vi "以太网测试界面.vi"() -> ()   [LabVIEW 2010]
panel:
  out "结果":bool
  out "接收数据":u32
  in  "发送数据":u32
  in  "btn_关闭":bool
  in  "btn_开始测试":bool
  # "以太网测试"
  # "输入数据："
  # "反馈数据："
  # "测试结果："
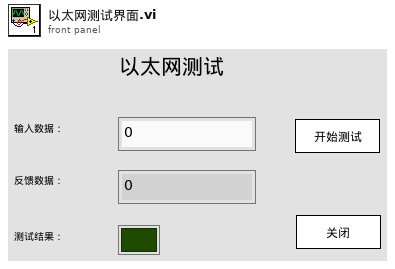
[diagram p1: front panel]
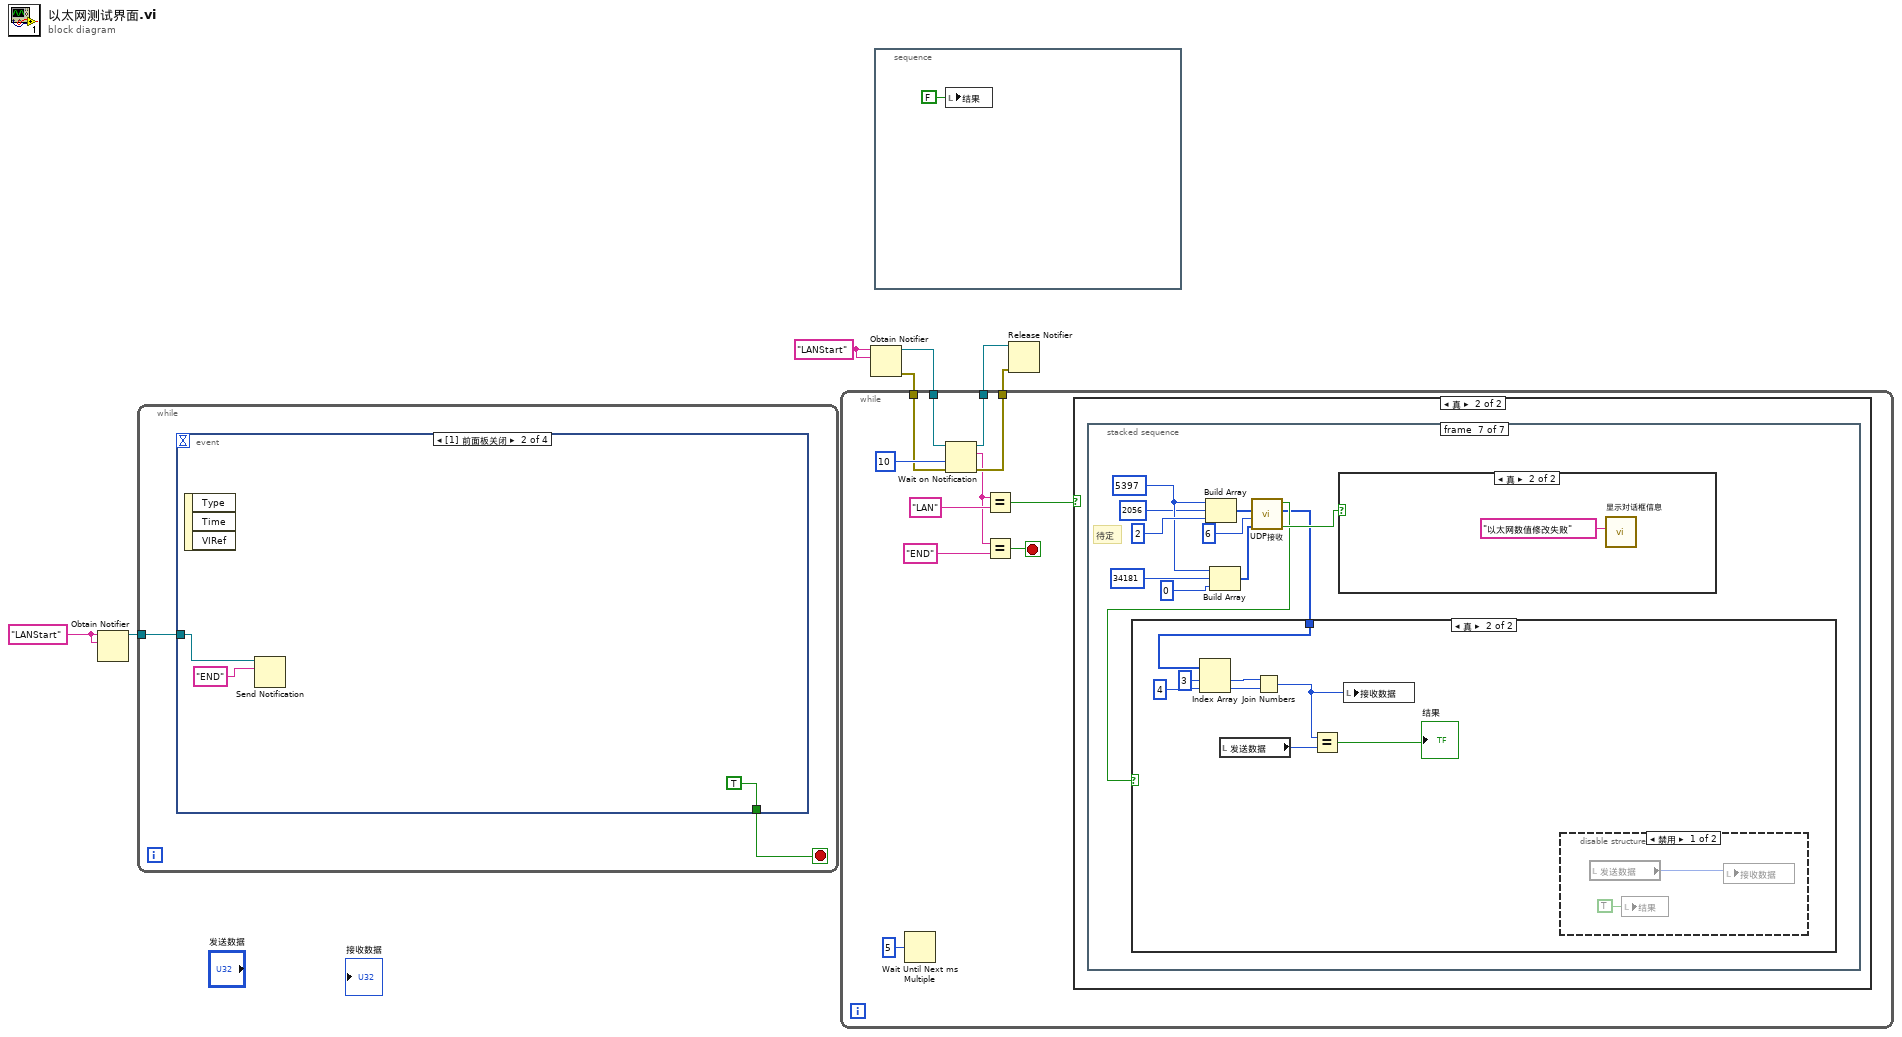
[diagram p0: block diagram]
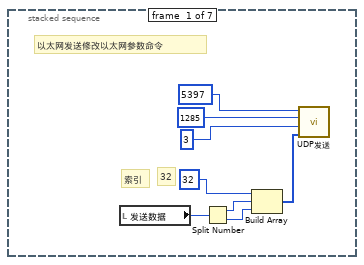
[diagram p3: hidden frame]
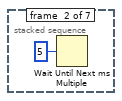
[diagram p4: hidden frame]
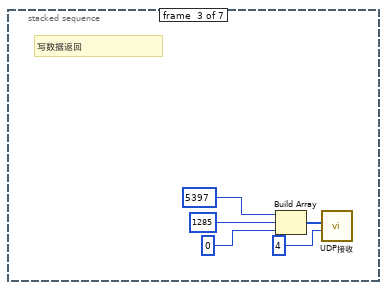
[diagram p5: hidden frame]
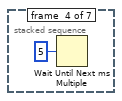
[diagram p6: hidden frame]
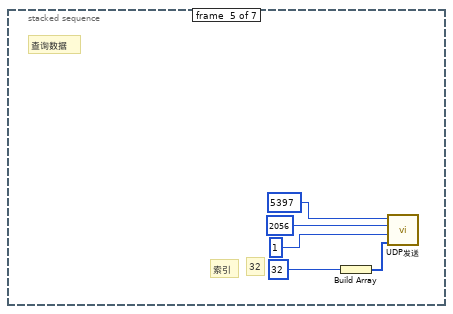
[diagram p7: hidden frame]
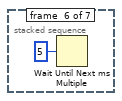
[diagram p8: hidden frame]
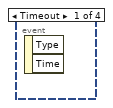
[diagram p12: hidden frame]
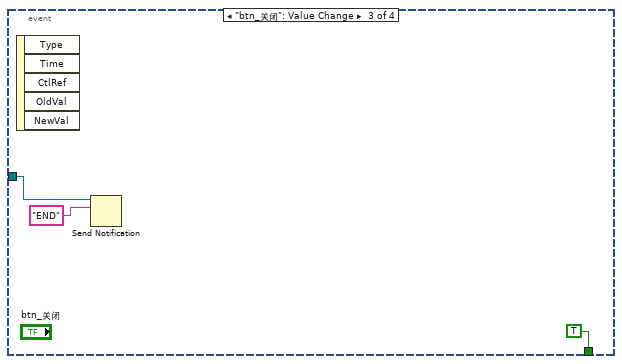
[diagram p13: hidden frame]
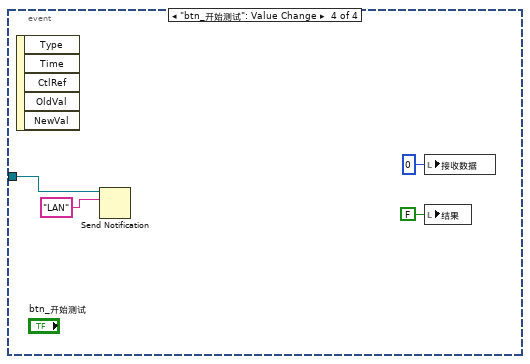
[diagram p14: hidden frame]
diagram:
  w2 = "LANStart" ("名称（未命名）")
  w5 = "LANStart" ("名称（未命名）")
  n1 = Obtain Notifier(name (unnamed)=w2, notification data type=w2) -> (notifier out=w1:refnum<notifier>)  [unwired: 2 in, 2 out]
  n2 = while {
    tunnel: w1 -> [w8]
    stop <- w9 stop-if-true
    n3 = event shown="[1] 前面板关闭" {
      selector: _ -> [_ _ _ _]
      dyn-events: _ -> [_ _ _ _]
      timeout: _ -> [_ _ _ _]
      tunnel: [_ TRUE TRUE _] -> w9
      tunnel: w8 -> [_ w10 w13 w18]
      event Timeout {
        n4 = event-data() -> ()  [unwired: 1 in, 2 out]
      }
      event Panel Close {
        n5 = event-data() -> ()  [unwired: 1 in, 3 out]
        n6 = Send Notification(notification="END" ("通知"), notifier=w10) -> ()  [unwired: 1 in, 2 out]
      }
      event "btn_关闭": Value Change {
        n7 = event-data() -> ()  [unwired: 1 in, 5 out]
        n8 = Send Notification(notification="END" ("通知"), notifier=w13) -> ()  [unwired: 1 in, 2 out]
      }
      event "btn_开始测试": Value Change {
        n9 = event-data() -> ()  [unwired: 1 in, 5 out]
        n10 = Send Notification(notification="LAN" ("通知"), notifier=w18) -> ()  [unwired: 1 in, 2 out]
        n11 = local write "接收数据"(u32 0 ("接收数据")) -> ()
        n12 = local write "结果"(FALSE ("结果")) -> ()
      }
    }
  }
  n13 = Obtain Notifier(name (unnamed)=w5, notification data type=w5) -> (notifier out=w7:refnum<notifier>, error out=w6:errorcluster)  [unwired: 2 in, 1 out]
  n14 = while {
    tunnel: w7 -> [w27]
    tunnel: w6 -> [w26]
    tunnel: [w25] -> w4
    tunnel: [w24] -> w3
    stop <- w20 stop-if-true
    n15 = Wait Until Next ms Multiple(millisecond multiple=u32 5 ("毫秒倍数")) -> ()  [unwired: 1 out]
    n16 = Wait on Notification(notifier=w27, timeout in ms (-1)=10 ("超时毫秒(-1)"), error in (no error)=w26) -> (notifier out=w25:refnum<notifier>, notification=w21:string, error out=w24:errorcluster)  [unwired: 1 in, 1 out]
    n17 = Equal?(x=w21, y="LAN" ("通知")) -> (x = y?=w22:bool)
    n18 = Equal?(x=w21, y="END" ("通知")) -> (x = y?=w20:bool)
    n19 = case shown="真" w22 {
      frame False {
      }
      frame True {
        n20 = stacked-sequence {
          frame #0 {
            # "32"
            # "以太网发送修改以太网参数命令"
            # "索引"
            n21 = local read "发送数据"() -> (w35:u32)
            n22 = Split Number(x=w35) -> (hi(x)=w33:u16, lo(x)=w32:u16)
            n23 = Build Array(u16 32, w33, w32) -> (w31:u16[])
            n24 = call "UDP发送.vi"("发送数据"=w31, "数据区字长"=u16 3, "报文类型"=u16 1285, "发送方标识"=u16 5397) -> ()  [unwired: 6 in, 1 out]
          }
          frame #1 {
            n25 = Wait Until Next ms Multiple(millisecond multiple=u32 5 ("毫秒倍数")) -> ()  [unwired: 1 out]
          }
          frame #2 {
            # "写数据返回"
            n26 = Build Array(u16 5397, u16 1285, u16 0) -> (w42:u16[])
            n27 = call "UDP接收.vi"("长度"=u16 4, "匹配帧信息_正常"=w42) -> ()  [unwired: 6 in, 4 out]
          }
          frame #3 {
            n28 = Wait Until Next ms Multiple(millisecond multiple=u32 5 ("毫秒倍数")) -> ()  [unwired: 1 out]
          }
          frame #4 {
            # "查询数据"
            # "32"
            # "索引"
            n29 = Build Array(u16 32) -> (w46:u16[])
            n30 = call "UDP发送.vi"("发送数据"=w46, "数据区字长"=u16 1, "报文类型"=u16 2056, "发送方标识"=u16 5397) -> ()  [unwired: 6 in, 1 out]
          }
          frame #5 {
            n31 = Wait Until Next ms Multiple(millisecond multiple=u32 5 ("毫秒倍数")) -> ()  [unwired: 1 out]
          }
          frame #6 {
            w59 = u16 5397
            # "待定"
            n32 = Build Array(w59, u16 2056, u16 2) -> (w57:u16[])
            n33 = Build Array(w59, u16 34181, u16 0 ("元素")) -> (w61:u16[])
            n34 = call "UDP接收.vi"("匹配帧信息_异常"=w61, "长度"=u16 6, "匹配帧信息_正常"=w57) -> ("异常_找到?"=w55:bool, "接收的一帧数据"=w53:u16[], "正常_找到?"=w54:bool)  [unwired: 5 in, 1 out]
            n35 = case shown="真" w54 {
              tunnel: w53 -> [_ w70]
              frame False {
              }
              frame True {
                n36 = Index Array(array=w70, index #1=3 ("索引"), index #2=4 ("索引")) -> (element #1=w64:u16, element #2=w63:u16)
                n37 = local read "发送数据"() -> (w66:u32)
                n38 = Join Numbers(hi=w64, lo=w63) -> ((hi.lo)=w67:u32)
                n39 = Equal?(x=w67, y=w66) -> (x = y?=→"结果":bool)
                n40 = local write "接收数据"(w67) -> ()
                n41 = disable-structure shown="禁用" {
                  frame Disabled {
                    n42 = local read "发送数据"() -> (w72:u32)
                    n43 = local write "结果"(TRUE ("结果")) -> ()
                    n44 = local write "接收数据"(w72) -> ()
                  }
                  frame Enabled {
                  }
                }
              }
            }
            n45 = case shown="真" w55 {
              frame False {
              }
              frame True {
                n46 = call "显示对话框信息"("Message"="以太网数值修改失败") -> ()  [unwired: 9 in, 2 out]
              }
            }
          }
        }
      }
    }
  }
  n47 = stacked-sequence {
    frame #0 {
      n48 = local write "结果"(FALSE ("结果")) -> ()
    }
  }
  n49 = Release Notifier(notifier=w4, error in (no error)=w3) -> ()  [unwired: 1 in, 3 out]
